vi "Receive Message.vi"(8 "Error In":errorcluster, 11 "Data":variant) -> (0 "Error Out":errorcluster, 3 "Display Ref":refnum<vi>)   [LabVIEW 2023, in "Receiver.lvclass"]
doc: "The method receives the class data as variant and performs the over riding method and obtains the reference of the display VI."
uses:
  Receiver.lvclass
  Data/Data.lvclass
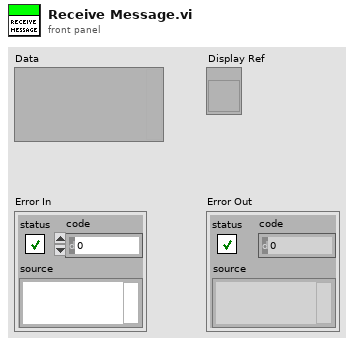
[diagram p1: front panel]
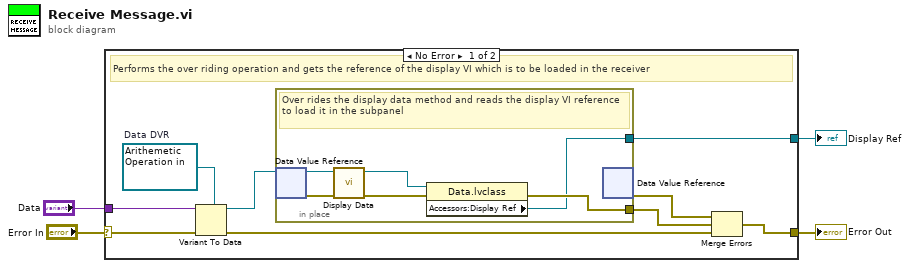
[diagram p0: block diagram]
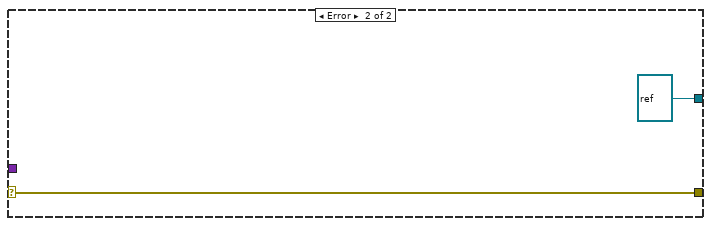
[diagram p2: hidden frame]
diagram:
  n1 = case shown="No Error" "Error In" {
    selector: "Error In" -> [w9 w21]
    tunnel: [w8 w21] -> w3
    tunnel: "Data" -> [w12 _]
    tunnel: [w5 refnum<vi> refnum ("Accessors:Display Ref")] -> w1
    frame No Error {
      w11 = refnum<data-value> refnum  # Data DVR
      # "Performs the over riding operation and gets the reference of the display VI which is to be loaded in the receiver"
      n2 = Variant To Data(error in=w9, type=w11, Variant=w12) -> (data=w10:refnum<data-value>, error out=w13:errorcluster)
      n3 = in-place {
        in-place-border: [w16] -> w7
        in-place-border: [w14] -> w5
        # "Over rides the display data method and reads the display VI reference to load it in the subpanel"
        n4 = in-place-dvr #1(w10) -> (w17:refnum<class "Data.lvclass">, w19:errorcluster)
        n5 = call-dynamic "Display Data.vi"("Error in"=w19, "Data in"=w17) -> ("Error Out"=w18:errorcluster, "Data out"=w15:refnum<class "Data.lvclass">)  [unwired: 8 in]
        n6 = property class="Data.lvclass"(reference=w15, error in=w18) -> (error out=w16:errorcluster, "Accessors:Display Ref"=w14:refnum<vi>)  [unwired: 1 out]
        n7 = in-place-dvr #1() -> (w6:errorcluster)  [unwired: 1 in, 1 out]
      }
      n8 = Merge Errors(w6, w7, w13) -> (w8:errorcluster)
    }
    frame Error {
    }
  }
  "Error Out" <- w3
  "Display Ref" <- w1
